vi "PopulateRegistersInfo.vi"(8 "error in (no error)":errorcluster, 11 "CameraDemo in":refnum<class "CameraDemo.lvclass">) -> (0 "error out":errorcluster, 3 "CameraDemo out":refnum<class "CameraDemo.lvclass">)   [LabVIEW 2020, in "CameraI2COUSB.lvlib" / "CameraDemo.lvclass"]
uses:
  CameraDemo.lvclass
  CameraDemo.lvclass/CameraDemo.ctl
  TypeDef/RegisterName.ctl
  TypeDef/RegisterInfo.ctl
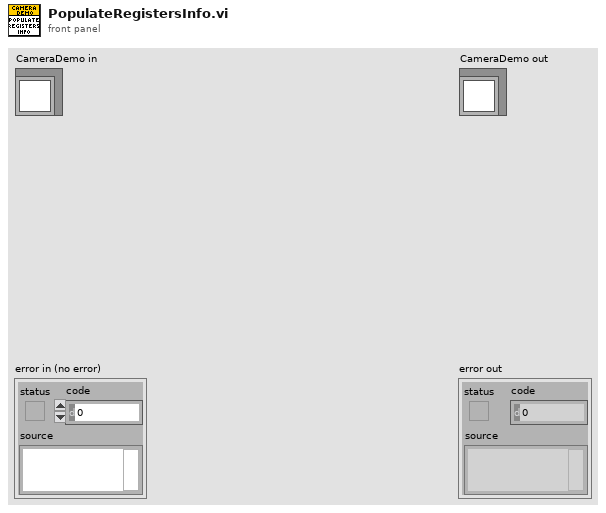
[diagram p1: front panel]
types:
  T1 = typedef "CameraI2COUSB.lvlib/CameraDemo.lvclass/RegisterName.ctl" = enum16{"Clock Rate", "Frame Rate", "Image Type", "Resolution", "Snap", "Start Streaming", "Stop Streaming"}
  T2 = typedef "CameraI2COUSB.lvlib/CameraDemo.lvclass/RegisterInfo.ctl" = cluster{"Address":u16, "Lenght":u32}
  T3 = cluster{"Register Name":T1, "Register Info":T2}[]
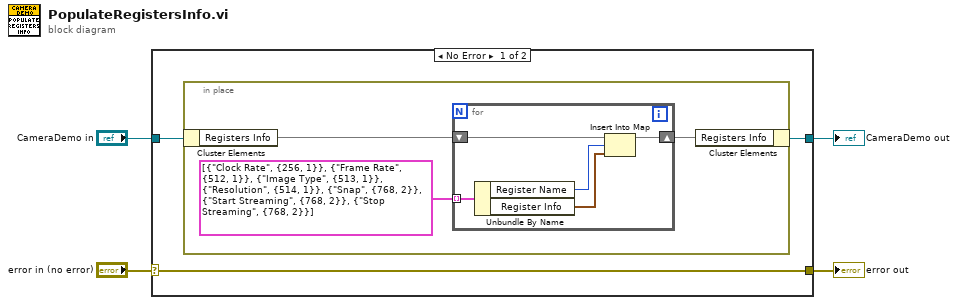
[diagram p0: block diagram]
diagram:
  n1 = case shown="No Error" "error in (no error)" {
    selector: "error in (no error)" -> [w5 w17]
    tunnel: [w5 w17] -> w3
    tunnel: [w6 w16] -> w1
    tunnel: "CameraDemo in" -> [w7 w16]
    frame No Error {
      n2 = in-place {
        n3 = in-place-cluster #1(w7) -> ("Registers Info"=w10:map{T1, T2})
        n4 = for {
          shift-right: [w14] -> w8
          shift-left: w10 -> [w15]
          tunnel: T3 [{"Register Name"=enum."Clock Rate", "Register Info"={"Address"=256, "Lenght"=1}}, {"Register Name"=enum."Frame Rate", "Register Info"={"Address"=512, "Lenght"=1}}, {"Register Name"=enum."Image Type", "Register Info"={"Address"=513, "Lenght"=1}}, {"Register Name"=enum."Resolution", "Register Info"={"Address"=514, "Lenght"=1}}, {"Register Name"=enum."Snap", "Register Info"={"Address"=768, "Lenght"=2}}, {"Register Name"=enum."Start Streaming", "Register Info"={"Address"=768, "Lenght"=2}}, {"Register Name"=enum."Stop Streaming", "Register Info"={"Address"=768, "Lenght"=2}}] -> [w13] mode=indexing
          n5 = Unbundle By Name(w13) -> ("Register Name"=w12:T1, "Register Info"=w11:T2)
          n6 = Insert Into Map(map in=w15, key=w12, value=w11) -> (map out=w14:map{T1, T2})  [unwired: 2 out]
        }
        n7 = in-place-cluster #1("Registers Info"=w8) -> (w6:refnum<class "CameraDemo.lvclass">)
      }
    }
    frame Error {
    }
  }
  "error out" <- w3
  "CameraDemo out" <- w1
